vi "Pagina manutenzione avvio.vi"() -> ()   [LabVIEW 2022 SP3]
uses:
  Labview/Globali.vi
  <vilib>/Utility/file.llb/Read From Spreadsheet File (string).vi
  <vilib>/Utility/file.llb/Write To Spreadsheet File (string).vi
panel:
  in  "stop":bool
  out "Array 3":bool[](array[boolean])
  in  "Tabella manutenzioni":T1(array[cluster])
  out "Prossimo controllo":string
  out "Ultimo controllo":string="ULTIMO CONTROLLO"
  out "Tipo controllo":string="TIPO INTERVENTO"
  out "Tipo pagina":string="PAGINA MANUTENZIONE"
  out "Indicazioni":string="Operatore:\t\t\t\t\t\t\t\t\t\t\t\t\t\t\t\toperatore\t\t\t\t\t\t\t\t\t\t\t\t\t\t\t\tPart number:\t\t\t\t\t\t\t\t\t\t\t\t\t\t\t\t60159655\t\t\t\t\t\t\t\t\t\t\t\t\t\t\t\tMatricola:\t\t\t\t\t\t\t\t\t\t\t\t\t\t\t\t4234\t\t\t\t\t\t\t\t\t\t\t\t\t\t\t\tStatus \t\t\t\t\t\t\t\t\t\t\t\t\t\t\t\tC:\\Documents and Settings\\IVECO\\Reports\\AAT3000 2° - 60159655\\Produzione"
  out "Picture":picture
  out "Versione SW":dbl=2.0 format="%.2f"
  out "Linea":string="BANCO PROVA TENUTA"
  out "Testo allarmi":string caption="ALLARMI"
  out "Testo fase collaudo":string caption="FASE COLLAUDO"
  out "Testo segnalazioni":string caption="SEGNALAZIONI"
  out "Testo messaggi":string caption="MESSAGGI"
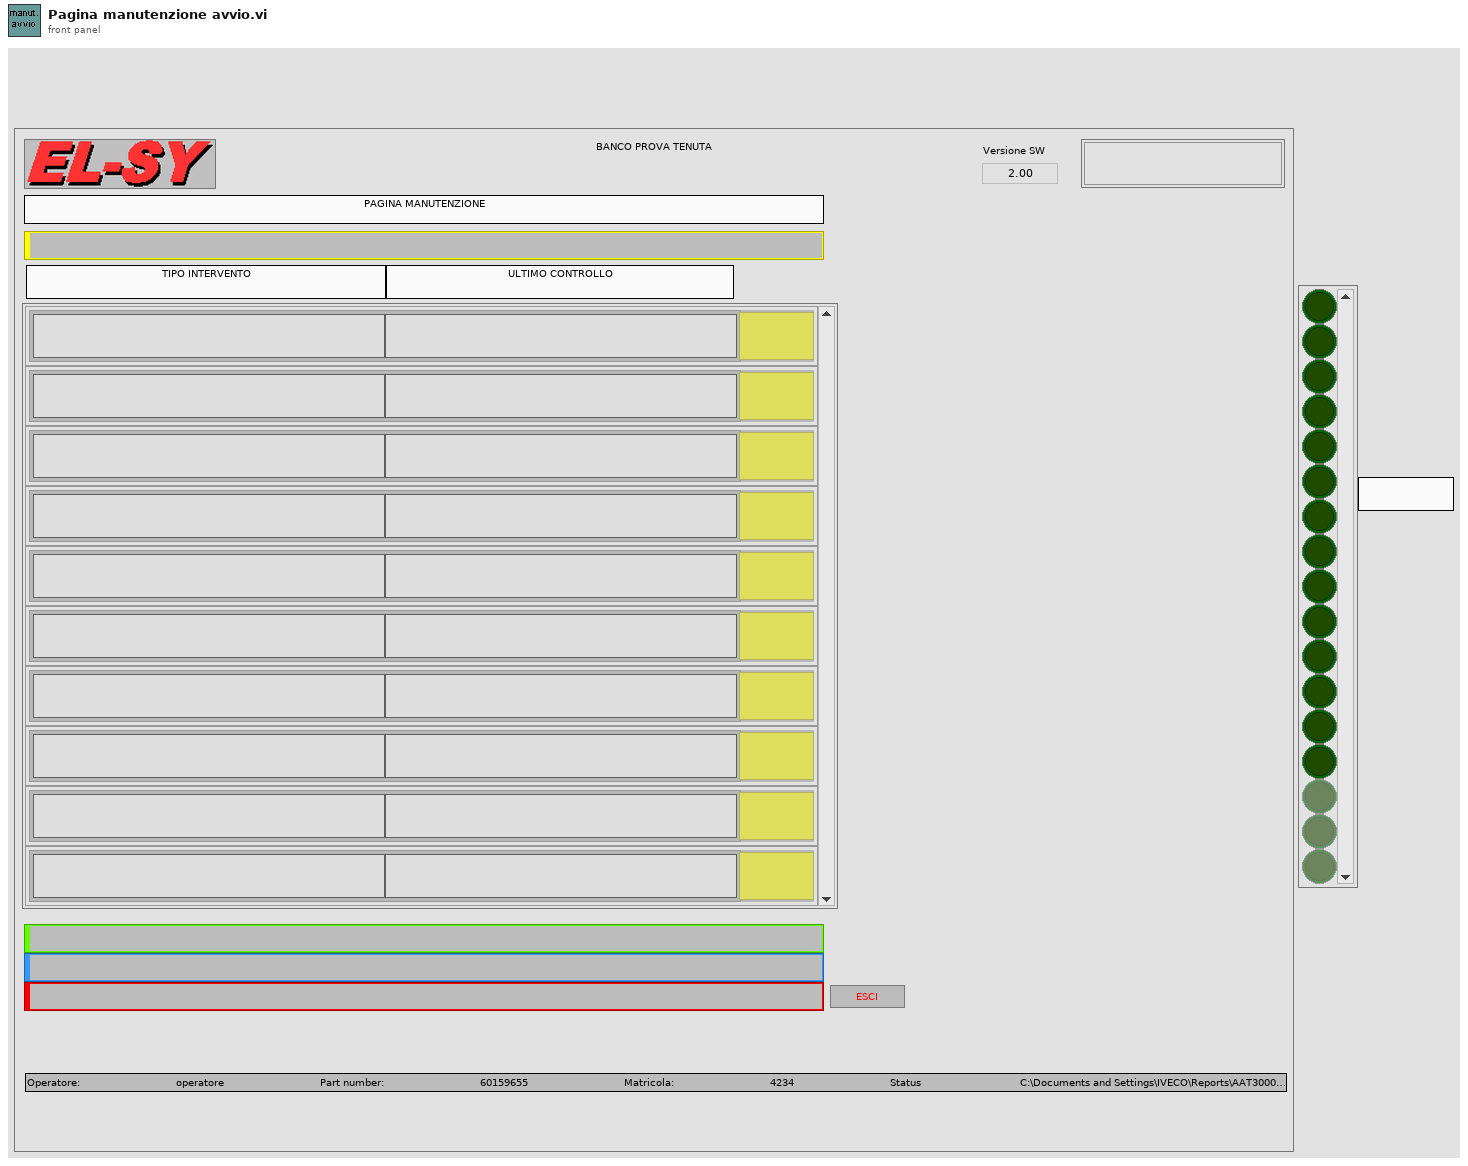
[diagram p1: front panel]
types:
  T1 = cluster{"Operazione":string[], "Eseguito":bool}[]
  T2 = cluster{"appended array":string[], "Eseguito":bool}
  T3 = cluster{"appended array":string[], "Eseguito":bool}[]
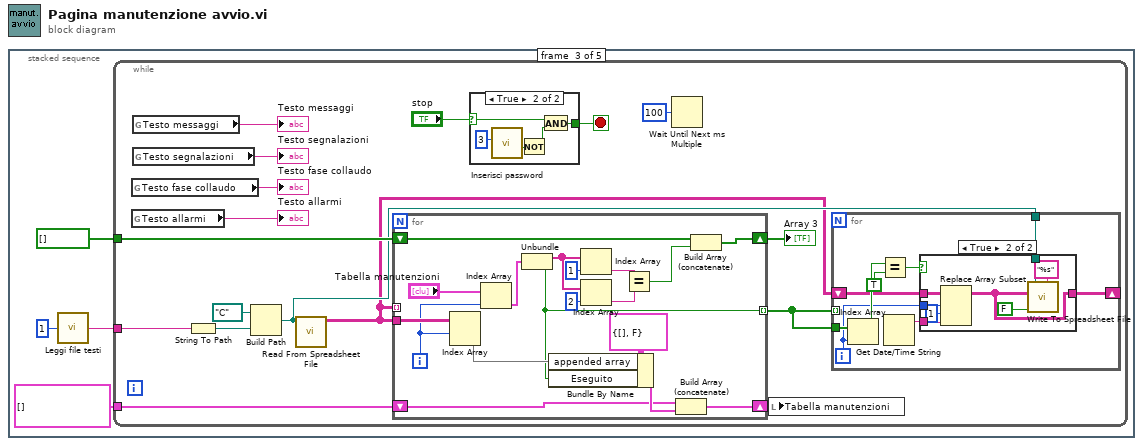
[diagram p0: block diagram]
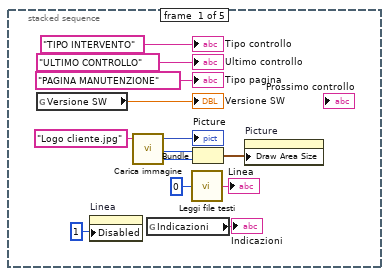
[diagram p2: hidden frame]
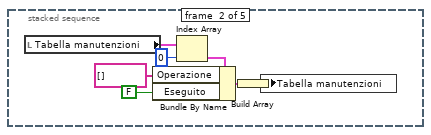
[diagram p3: hidden frame]
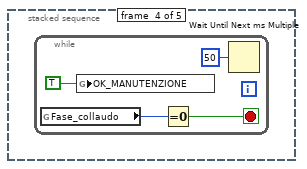
[diagram p6: hidden frame]
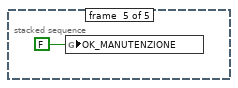
[diagram p7: hidden frame]
diagram:
  n1 = stacked-sequence {
    frame #0 {
      n2 = global read "Globali.vi" "Versione SW"() -> (→"Versione SW":dbl)
      n3 = property on="Linea" class="Str"("Disabled"=u8 1) -> ()  [unwired: 2 in, 2 out]
      n4 = call "Carica immagine.vi"("Immagine JPG"="Logo cliente.jpg") -> ("altezza"=w5:i16, "larghezza"=w4:i16, "Picture"=→"Picture":picture)  [unwired: 2 in]
      n5 = global read "Globali.vi" "Indicazioni"() -> (→"Indicazioni":string)
      n6 = call "Leggi file testi.vi"("Numero riga"=0) -> ("Testo"=→"Linea":string)  [unwired: 3 in, 1 out]
      n7 = Bundle("larghezza"=w4, "altezza"=w5) -> (w6:cluster{"larghezza":i16, "altezza":i16})  [unwired: 1 in]
      n8 = property on="Picture" class="Pict"("Draw Area Size"=w6) -> ()  [unwired: 2 in, 2 out]
      "Tipo pagina" <- "PAGINA MANUTENZIONE" ("Tipo pagina")
      "Tipo controllo" <- "TIPO INTERVENTO" ("Tipo controllo")
      "Ultimo controllo" <- "ULTIMO CONTROLLO" ("Ultimo controllo")
    }
    frame #1 {
      n9 = local read "Tabella manutenzioni"() -> (w15:T1)
      n10 = Index Array(array=w15, index=0) -> (element=w17:cluster{"Operazione":string[], "Eseguito":bool})
      n11 = Bundle By Name(cluster=w17, "Operazione"=string[] [], "Eseguito"=FALSE) -> (w19:cluster{"Operazione":string[], "Eseguito":bool})
      n12 = Build Array(w19) -> (w20:T1)
      n13 = local write "Tabella manutenzioni"(w20) -> ()
    }
    frame #2 {
      n14 = call "Leggi file testi.vi"("Numero riga"=1) -> ("Testo"=w23:string)  [unwired: 3 in, 1 out]
      n15 = while {
        tunnel: w23 -> [w36]
        tunnel: T1 [] ("Tabella manutenzioni 2") -> [w33]
        tunnel: bool[] [] -> [w32]
        stop <- w27 stop-if-true
        n16 = global read "Globali.vi" "Testo fase collaudo"() -> (→"Testo fase collaudo":string)
        n17 = global read "Globali.vi" "Testo allarmi"() -> (→"Testo allarmi":string)
        n18 = global read "Globali.vi" "Testo messaggi"() -> (→"Testo messaggi":string)
        n19 = global read "Globali.vi" "Testo segnalazioni"() -> (→"Testo segnalazioni":string)
        n20 = String To Path(string=w36) -> (path=w35:path)
        n21 = Build Path(base path=path "C:/", name or relative path=w35) -> (appended path=w26:path)
        n22 = call-poly <vilib>:"Read From Spreadsheet File.vi"("file path (dialog if empty)"=w26) -> ("all rows"=w25:string[][])  [unwired: 6 in, 4 out]
        n23 = for {
          tunnel: w25 -> [w70]
          tunnel: w25 -> [_] mode=indexing
          shift-right: [w82] -> w30
          shift-left: w33 -> [w81]
          shift-right: [w73] -> w31
          shift-left: w32 -> [w72]
          tunnel: [w66] -> w29 mode=indexing
          i -> [w69]
          n24 = Index Array(array=w70, index (row)=w69) -> (element=w67:string[])  [unwired: 1 in]
          n25 = Index Array(array="Tabella manutenzioni", index=w69) -> (element=w68:cluster{"Operazione":string[], "Eseguito":bool})
          n26 = Unbundle(w68) -> ("Operazione"=w77:string[], "Eseguito"=w66:bool)
          n27 = Bundle By Name(cluster=T2 {"appended array"=[], "Eseguito"=FALSE}, "appended array"=w67, "Eseguito"=w66) -> (w83:T2)
          n28 = Index Array(array=w77, index=1) -> (element=w76:string)
          n29 = Index Array(array=w77, index=2) -> (element=w75:string)
          n30 = Equal?(x=w76, y=w75) -> (x = y?=w74:bool)
          n31 = Build Array (concatenate)(w81, w83) -> (w82:T3)
          n32 = Build Array (concatenate)(w72, w74) -> (w73:bool[])
        }
        "Array 3" <- w31
        n33 = case shown="True" "stop" {
          selector: "stop" -> [w42 w45]
          tunnel: [w42 w43] -> w27
          frame False {
          }
          frame True {
            n34 = call "Inserisci password.vi"("Livello pass"=3) -> ("Annulla?"=w46:bool)  [unwired: 10 in]
            n35 = Not(x=w46) -> (.not. x?=w44:bool)
            n36 = And(x=w45, y=w44) -> (x .and. y?=w43:bool)
          }
        }
        n37 = Wait Until Next ms Multiple(millisecond multiple=u32 100) -> ()  [unwired: 1 out]
        n38 = local write "Tabella manutenzioni"(w30) -> ()
        n39 = for {
          tunnel: w29 -> [w55]
          tunnel: w29 -> [_] mode=indexing
          tunnel: w26 -> [w50]
          shift-right: [w48] -> _
          shift-left: w25 -> [w49]
          i -> [w51]
          n40 = Index Array(array=w55, index=w51) -> (element=w53:bool)
          n41 = Equal?(x=w53, y=TRUE) -> (x = y?=w52:bool)
          n42 = Get Date/Time String() -> (date string=w56:string)  [unwired: 3 in, 1 out]
          n43 = case shown="True" w52 {
            tunnel: w49 -> [w57 w65]
            tunnel: w51 -> [_ w64]
            tunnel: w56 -> [_ w63]
            tunnel: w50 -> [_ w59]
            tunnel: [w57 w58] -> w48
            frame False {
            }
            frame True {
              n44 = Replace Array Subset(array=w65, new element=w63, index (row)=w64, index (col)=1 ("disabled index (col)")) -> (w58:string[][])
              n45 = call-poly <vilib>:"Write To Spreadsheet File.vi"("format (%s)"="%s" ("format (%.3f)"), "append to file? (new file:F)"=FALSE, "2D data"=w58, "file path (dialog if empty)"=w59) -> ()  [unwired: 4 in, 1 out]
            }
          }
        }
      }
    }
    frame #3 {
      n46 = while {
        stop <- w85 stop-if-true
        n47 = global read "Globali.vi" "Fase_collaudo"() -> (w86:u16)
        n48 = global write "Globali.vi" "OK_MANUTENZIONE"(TRUE ("OK_MANUTENZIONE")) -> ()
        n49 = Equal To 0?(x=w86) -> (x = 0?=w85:bool)
        n50 = Wait Until Next ms Multiple(millisecond multiple=u32 50) -> ()  [unwired: 1 out]
      }
    }
    frame #4 {
      n51 = global write "Globali.vi" "OK_MANUTENZIONE"(FALSE ("OK_MANUTENZIONE")) -> ()
    }
  }
